vi "Save_Pulse.vi"(2 "error in":errorcluster, 3 "Pulse sequence":T1[](array[typedef]) {"channel" min=2 max=13 step=1}, 4 "Filename (.ini)":string="Config_Ver_1\\pulse_sequence.ini") -> (0 "error out":errorcluster)   [LabVIEW 2021]
uses:
  Drivers/Arduino_Pulse_Generator/Configurate/Channel_Pulse_Stream.ctl
  Pulse_Sequence_Global.vi
  <vilib>/Utility/config.llb/Write Key (String).vi
  <vilib>/Utility/config.llb/NI_LVConfig.lvlib
panel:
  # "Remember that config files are .ini, \nconfig file will be save in ...\\Config_Files\\(filename).ini"
  # "One can easily add files into folder placed inside ...\\Config_Files\\ (folder)\nby writing Filename as (folder)\\(filename).ini, but firstly one have to manualy\ncreate that folder"
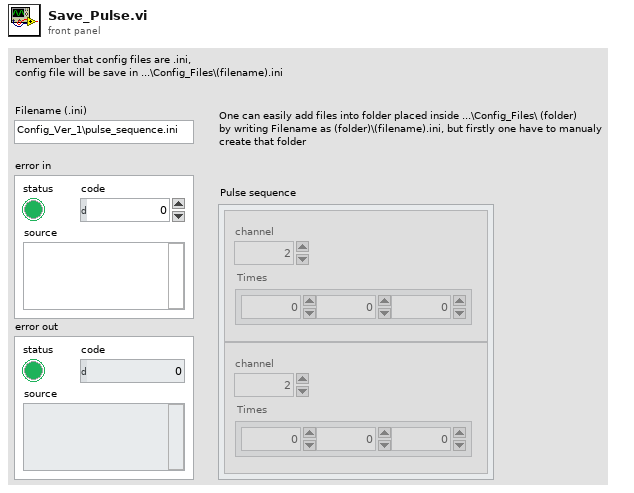
[diagram p1: front panel]
types:
  T1 = typedef "Channel_Pulse_Stream.ctl" = cluster{"Times":dbl[], "channel":u8}
  T2 = typedef "NI_LVConfig.lvlib/Config Data RefNum.ctl" = refnum<k1>
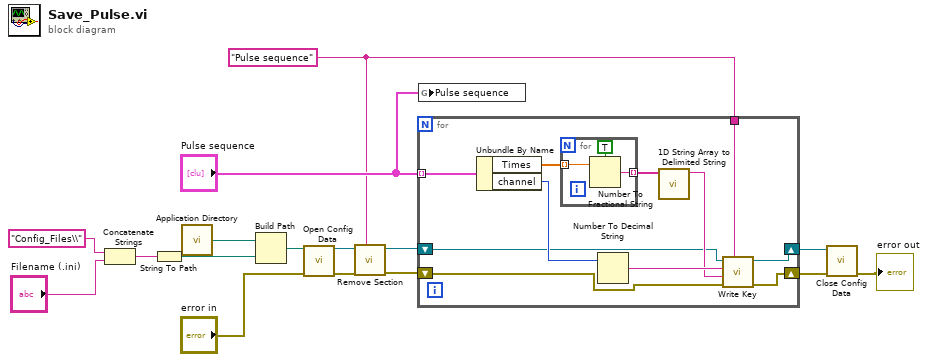
[diagram p0: block diagram]
diagram:
  w4 = "Pulse sequence" ("section")
  n1 = Concatenate Strings("Config_Files\\" ("string"), "Filename (.ini)") -> (w10:string)
  n2 = String To Path(string=w10) -> (path=w13:path)
  n3 = call <vilib>:"Application Directory.vi"() -> ("Application Directory"=w16:path)
  n4 = Build Path(base path=w16, name or relative path=w13) -> (appended path=w15:path)
  n5 = call <vilib>:"Open Config Data.vi"("error in (no error)"="error in", "configuration file path"=w15) -> ("error out"=w2:errorcluster, "refnum"=w3:T2)  [unwired: 7 in, 1 out]
  n6 = call <vilib>:"Remove Section.vi"("section"=w4, "error in (no error)"=w2, "refnum"=w3) -> ("error out"=w1:errorcluster, "refnum out"=w5:T2)  [unwired: 6 in, 1 out]
  n7 = for {
    tunnel: "Pulse sequence" -> [w27] mode=indexing
    shift-right: [w18] -> w8
    shift-left: w5 -> [w21]
    shift-right: [w19] -> w7
    shift-left: w1 -> [w20]
    tunnel: w4 -> [w17]
    n8 = Unbundle By Name(w27) -> ("Times"=w26:dbl[], "channel"=w24:u8)
    n9 = for {
      tunnel: w26 -> [w30] mode=indexing
      tunnel: [w29] -> w25 mode=indexing
      n10 = Number To Fractional String(use system decimal point (T)=TRUE, number=w30) -> (F-format string=w29:string)  [unwired: 2 in]
    }
    n11 = Number To Decimal String(number=w24) -> (decimal integer string=w23:string)  [unwired: 1 in]
    n12 = call <vilib>:"1D String Array to Delimited String.vi"("string array"=w25) -> ("delimited string"=w22:string)  [unwired: 10 in]
    n13 = call-poly <vilib>:"Write Key.vi"("section"=w17, "error in (no error)"=w20, "value"=w22, "key"=w23, "refnum"=w21) -> ("error out"=w19:errorcluster, "refnum out"=w18:T2)  [unwired: 4 in, 1 out]
  }
  n14 = global write "Pulse_Sequence_Global.vi" "Pulse sequence"("Pulse sequence") -> ()
  n15 = call <vilib>:"Close Config Data.vi"("error in (no error)"=w7, "refnum"=w8) -> ("error out"=→"error out":errorcluster)  [unwired: 8 in, 1 out]
